vi "AutoIsTwoBall.vi"(11 "AutoMode":T1) -> (3 "IsTwoBall?":bool)   [LabVIEW 2013]
doc: "Determines if autonomous should do one or two balls, as implied from the AutoMode."
uses:
  AutoMode.ctl
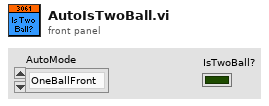
[diagram p1: front panel]
types:
  T1 = typedef "AutoMode.ctl" = enum16{"OneBallFront", "OneBallCollector", "TwoBallNormal", "TwoBallHot"}
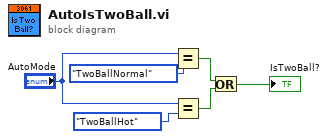
[diagram p0: block diagram]
diagram:
  n1 = Equal?(x="AutoMode", y=AutoMode."TwoBallNormal") -> (x = y?=w2:bool)
  n2 = Equal?(x="AutoMode", y=AutoMode."TwoBallHot") -> (x = y?=w3:bool)
  n3 = Or(x=w2, y=w3) -> (x .or. y?=→"IsTwoBall?":bool)
